vi "Library Append Text File.vi"(0 "file path":path, 1 "convert eol (F)":bool, 7 "text to write":string, 11 "error in (no error)":errorcluster) -> (4 "dup path":path, 15 "error out":errorcluster)   [LabVIEW 2012]
doc: "Writes a text file with optional eol conversion."
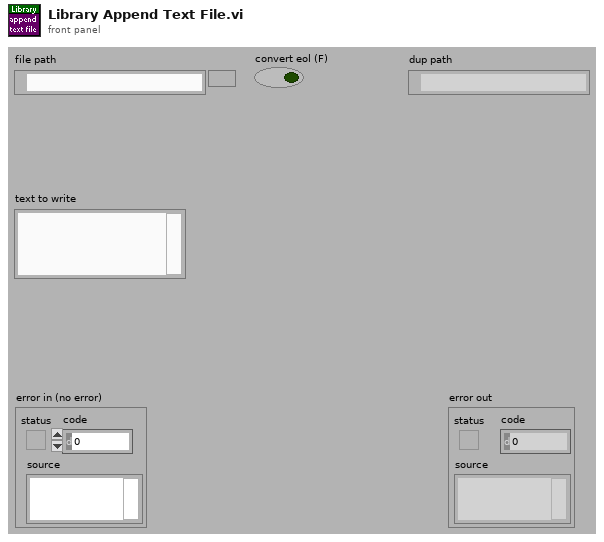
[diagram p1: front panel]
types:
  T1 = enum16{"deny read/write", "deny write-only", "deny none"}
  T2 = enum16{"read/write", "read-only", "write-only", "write-only (truncate)"}
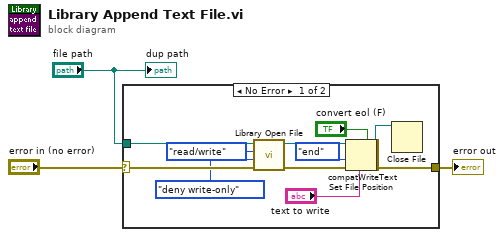
[diagram p0: block diagram]
diagram:
  n1 = case shown="No Error" "error in (no error)" {
    selector: "error in (no error)" -> [w15 w17]
    tunnel: [w16 w17] -> w3
    tunnel: "file path" -> [w8 _]
    frame No Error {
      n2 = call "Library Open File.vi"("error in (no error)"=w15, "deny mode (deny none)"=T1."deny write-only", "open mode (read/write)"=T2."read/write", "file path"=w8) -> ("error out"=w13:errorcluster, "refnum"=w14:refnum<file>)  [unwired: 2 in]
      n3 = Set File Position(refnum=w14, from (0:start)=enum16{"start", "end", "current"}."end" ("pos mode (0:2)"), error in=w13) -> (refnum out=w5:refnum<file>, error out=w4:errorcluster)  [unwired: 1 in]
      n4 = call <vilib>:"compatWriteText.vi"("convert eol (F)"="convert eol (F)", "data"="text to write", "error in"=w4, "refnum"=w5) -> ("error out"=w16:errorcluster, "dup refnum"=w10:refnum<file>)  [unwired: 6 in]
      n5 = Close File(refnum=w10) -> ()  [unwired: 1 in, 2 out]
    }
    frame Error {
    }
  }
  "error out" <- w3
  "dup path" <- "file path"
